vi "Test Cashier No Error Processing Order.vi"(8 "error in (no error)":errorcluster, 11 "Cashier Test in":refnum<class "Cashier Test.lvclass">) -> (0 "error out":errorcluster, 3 "Cashier Test out":refnum<class "Cashier Test.lvclass">)   [LabVIEW 2020, in "Cashier Test.lvclass"]
uses:
  Cashier Test.lvclass
  C:/Users/anton/Documents/GitHub/Triarc-Examples/Coffee Shop/Worker Test/Worker Test.lvclass
  C:/Program Files (x86)/National Instruments/LabVIEW 2020/vi.lib/Asteme/LUnit/Test Case.lvclass
  Support/Beverages/TypeDefs/Drink Type.ctl
  Support/Beverages/TypeDefs/Options.ctl
  Processes/People/Customers/Customer/Customer.lvclass
  <vilib>/Asteme/Triarc Framework Test Suite/Mock Error Handler/Mock Error Handler.lvclass
  C:/Program Files (x86)/National Instruments/LabVIEW 2020/vi.lib/Asteme/Triarc Framework/Error Handler Interface/Error Handler Interface.lvclass
  Test Doubles/Stub Job Handler/Stub Job Handler.lvclass
  C:/Users/anton/Documents/GitHub/Triarc-Examples/Coffee Shop/Process Job/Job Handler.lvclass
  <vilib>/Asteme/Triarc Framework/Process/Process.lvclass/Process.ctl
  <vilib>/Asteme/LUnit/Test Case.lvclass/Test Case.ctl
  <vilib>/Asteme/LUnit/LUnit Assertion Result.lvclass/LUnit Assertion Result.ctl
  <vilib>/Asteme/Triarc Framework/Process/Protected/Messaging/Enqueue Message.vi
  <vilib>/Asteme/Triarc Framework/Process/Public/Lifecycle/Get Lifecycle State.vi
  <vilib>/Asteme/Triarc Framework/Process/Private/SubVIs/Wait for finish.vi
  <vilib>/Asteme/Triarc Framework/Process/Private/SubVIs/Set Lifecycle State.vi
  <vilib>/Asteme/LUnit/Palette/Pass.vi
  <vilib>/Asteme/LUnit/Palette/Fail.vi
  <vilib>/Asteme/LUnit/Set Assertion Type.vi
  <vilib>/AdvancedString/1D String Array to Delimited String.vi
  <vilib>/Utility/error.llb/Clear Errors.vi
  <vilib>/Asteme/LUnit/Add test result.vi
  <vilib>/Asteme/LUnit/LUnit Write Passed.vi
  <vilib>/Asteme/LUnit/LUnit Get Test Case.vi
  <vilib>/Asteme/LUnit/Assertion Result/LUnit Get Test Name.vi
  <vilib>/Asteme/LUnit/LUnit Write Message.vi
  <vilib>/Asteme/LUnit/LUnit Write Description.vi
  <vilib>/Asteme/LUnit/LUnit Write Assertion Type.vi
  <vilib>/Asteme/LUnit/Read Test Case Name.vi
  Processes/People/Workers/Worker/Worker.lvclass
  C:/Program Files (x86)/National Instruments/LabVIEW 2020/vi.lib/Asteme/Triarc Framework/Process/Process.lvclass
  <vilib>/Utility/error.llb/Error Cluster From Error Code.vi
  <vilib>/Asteme/LUnit/LUnit Assertion Result.lvclass
  <vilib>/Asteme/Triarc Framework/Process/Process.lvclass
  Worker Test/Worker Test.lvclass
  Support/Order/Order.lvclass
  Support/Beverages/Beverage/Beverage.lvclass
  <vilib>/Asteme/LUnit/Test Case.lvclass
panel:
  out "Error":errorcluster
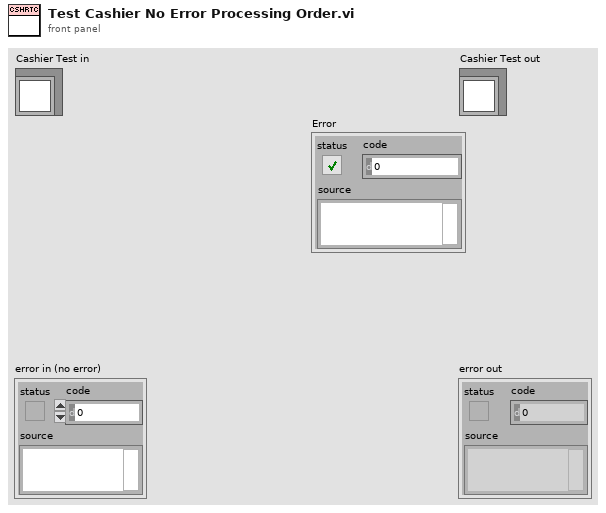
[diagram p1: front panel]
types:
  T1 = typedef "Beverage.lvclass/Drink Type.ctl" = enum16{"Dark Roast", "Decaf", "Espresso", "House Blend"}
  T2 = typedef "Beverage.lvclass/Options.ctl" = enum16{"<None>", "Milk", "Mocha", "Soy", "Whip"}
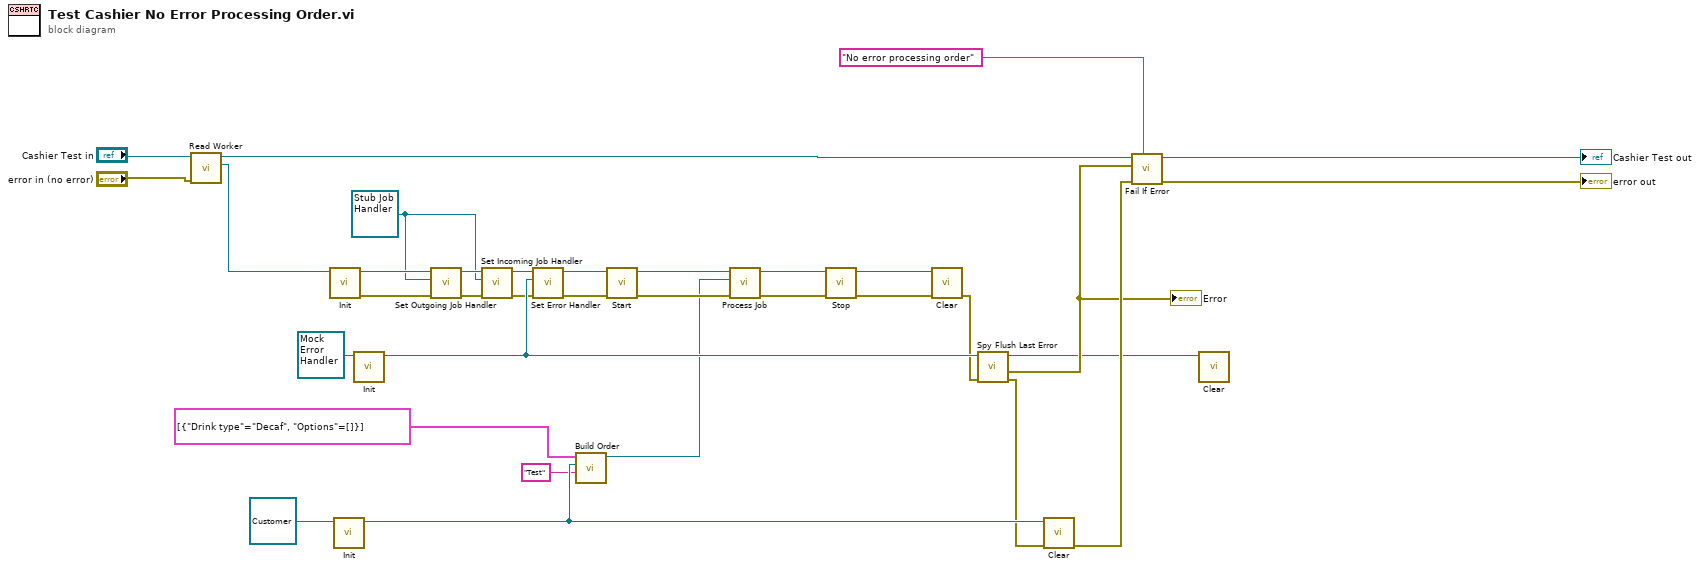
[diagram p0: block diagram]
diagram:
  w1 = refnum<class "Stub Job Handler.lvclass"> refnum ("Stub Job Processor.lvclass")
  n1 = call "Read Worker.vi"("error in (no error)"="error in (no error)", "Worker Test in"="Cashier Test in") -> ("Worker"=w22:refnum<class "Worker.lvclass">, "Worker Test out"=w21:refnum<class "Cashier Test.lvclass">)  [unwired: 7 in, 1 out]
  n2 = call-dynamic "Init.vi"("View In"=w22) -> ("error out"=w23:errorcluster, "View Out"=w6:refnum<class "Worker.lvclass">)  [unwired: 9 in]
  n3 = call-dynamic "Init.vi"("View In"=refnum<class "Customer.lvclass"> refnum ("Customer.lvclass")) -> ("View Out"=w18:refnum<class "Customer.lvclass">)  [unwired: 9 in, 1 out]
  n4 = call-dynamic "Init.vi"("Mock Error Handler In"=refnum<class "Mock Error Handler.lvclass"> refnum) -> ("Mock Error Handler Out"=w13:refnum<class "Mock Error Handler.lvclass">)  [unwired: 9 in, 1 out]
  n5 = call "Set Outgoing Job Handler.vi"("error in (no error)"=w23, "Work Dispatcher"=w1, "Worker In"=w6) -> ("error out"=w7:errorcluster, "Worker Out"=w4:refnum<class "Worker.lvclass">)  [unwired: 7 in]
  n6 = call "Set Incoming Job Handler.vi"("error in (no error)"=w7, "Job Handler"=w1, "Worker In"=w4) -> ("error out"=w5:errorcluster, "Worker Out"=w3:refnum<class "Worker.lvclass">)  [unwired: 7 in]
  n7 = call <vilib>:"Set Error Handler.vi"("error in (no error)"=w5, "Error Handler"=w13, "Process In"=w3) -> ("error out"=w16:errorcluster, "Process Out"=w15:refnum<class "Worker.lvclass">)  [unwired: 7 in]
  n8 = call "Build Order.vi"("Customer Name"="Test", "Customer"=w18, "Order"=cluster{"Drink type":T1, "Options":T2[]}[] [{"Drink type"=enum."Decaf", "Options"=[]}]) -> ("Order Out"=w8:refnum<class "Order.lvclass">)  [unwired: 7 in, 1 out]
  n9 = call <vilib>:"Start.vi"("error in (no error)"=w16, "Process In"=w15) -> ("error out"=w26:errorcluster, "Process Out"=w28:refnum<class "Worker.lvclass">)  [unwired: 8 in]
  n10 = call-dynamic "Process Job.vi"("error in (no error)"=w26, "Job"=w8, "Worker In"=w28) -> ("error out"=w30:errorcluster, "Worker Out"=w29:refnum<class "Worker.lvclass">)  [unwired: 7 in]
  n11 = call <vilib>:"Stop.vi"("error in (no error)"=w30, "Process In"=w29) -> ("error out"=w25:errorcluster, "Process Out"=w24:refnum<class "Worker.lvclass">)  [unwired: 7 in, 1 out]
  n12 = call-dynamic "Clear.vi"("error in (no error)"=w25, "View In"=w24) -> ("error out"=w12:errorcluster)  [unwired: 9 in]
  n13 = call <vilib>:"Spy Flush Last Error.vi"("error in (no error)"=w12, "Mock Error Handler In"=w13) -> ("error out"=w10:errorcluster, "Error"=w11:errorcluster, "Mock Error Handler Out"=w9:refnum<class "Mock Error Handler.lvclass">)  [unwired: 7 in]
  "Error" <- w11
  n14 = call-dynamic "Clear.vi"("error in (no error)"=w10, "View In"=w18) -> ("error out"=w17:errorcluster)  [unwired: 9 in]
  n15 = call <vilib>:"Fail If Error.vi"("Description"="No error processing order", "error in (no error)"=w17, "Assert error"=w11, "Test Case In"=w21) -> ("error out"=→"error out":errorcluster, "Test Case Out"=→"Cashier Test out":refnum<class "Cashier Test.lvclass">)  [unwired: 6 in]
  n16 = call-dynamic "Clear.vi"("Mock Process In"=w9) -> ()  [unwired: 10 in, 1 out]
